vi "坐标变换.vi"(11 "数组":string[](array[string])) -> (2 "数组 2":cluster{"字符串":i32, i32}[](array[cluster]))   [LabVIEW 2013]
panel:
  out "数字":i32[](array[numeric])
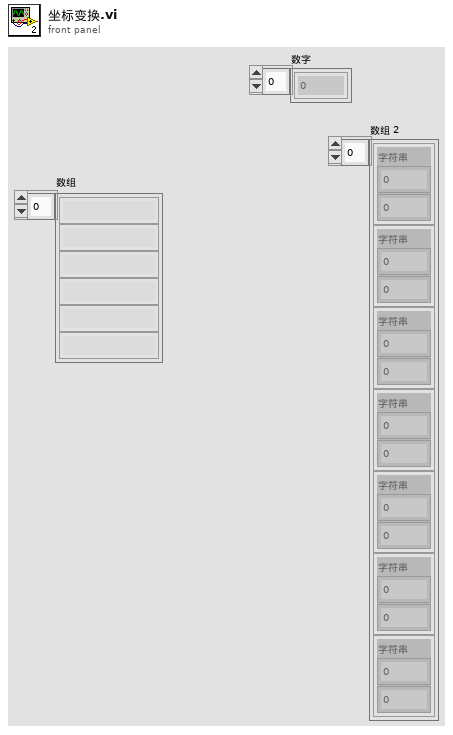
[diagram p1: front panel]
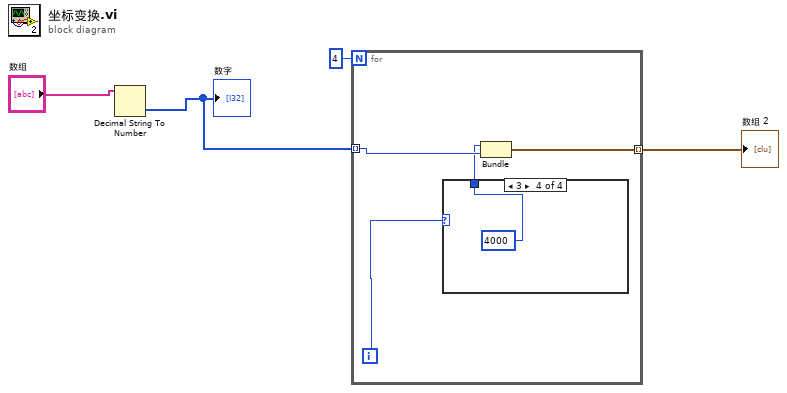
[diagram p0: block diagram]
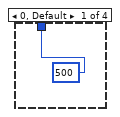
[diagram p2: hidden frame]
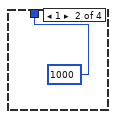
[diagram p3: hidden frame]
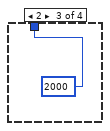
[diagram p4: hidden frame]
diagram:
  n1 = Decimal String To Number(string="数组") -> (number=w3:i32[])  [unwired: 2 in, 1 out]
  "数字" <- w3
  n2 = for {
    N: 4 -> [_]
    tunnel: w3 -> [w7] mode=indexing
    tunnel: [w8] -> w1 mode=indexing
    i -> [w6]
    n3 = case shown="3" w6 {
      tunnel: [500 1000 2000 4000] -> w5
      frame 0, Default {
      }
      frame 1 {
      }
      frame 2 {
      }
      frame 3 {
      }
    }
    n4 = Bundle(w5, "字符串"=w7) -> (w8:cluster{i32, "字符串":i32})  [unwired: 1 in]
  }
  "数组 2" <- w1
